vi "closeDevices.vi"(8 "Erreur d'entrée DAS":errorcluster caption="Error in", 9 "ID a l'entrée":T1, 10 "Erreur d'entrée alim":errorcluster caption="Error in", 11 "Device information in":string[](array[string])) -> (0 "Erreur de sortie":errorcluster caption="valeur sélectionnée", 1 "TCP/IP Settings:Dot-Notation Address":string)   [LabVIEW 2019]
doc: "Il ferme tous les connections avec les machines."
uses:
  <instrlib>/Sefram DAS240/Sefram DAS240.lvlib
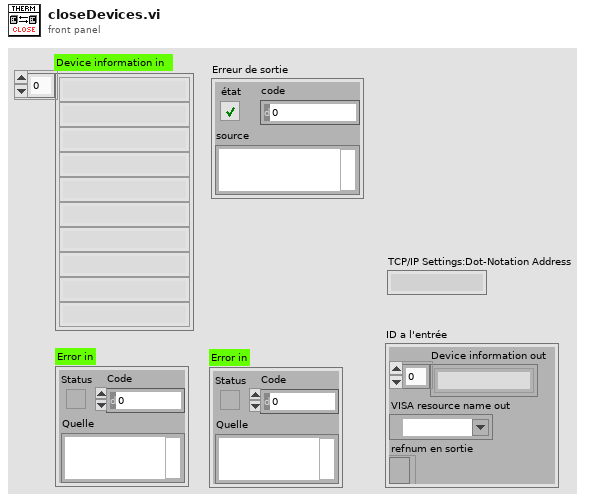
[diagram p1: front panel]
types:
  T1 = cluster{"Device information out":string[], "VISA resource name out":refnum<visa-resource-name>, "refnum en sortie":refnum<file>}
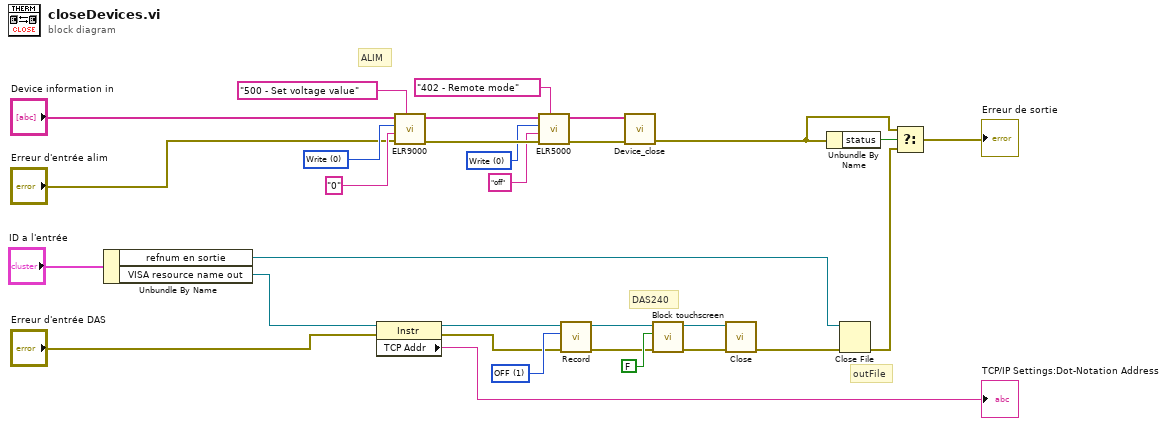
[diagram p0: block diagram]
diagram:
  w13 = u16 1 items=["ON", "OFF", "TRIG"] ("Record State")
  w21 = u8 0 items=["Write", "Read"] ("Access")
  w26 = u8 0 items=["Write", "Read"] ("Access")
  # "outFile"
  # "DAS240"
  # "ALIM"
  n1 = Unbundle By Name("ID a l'entrée") -> ("refnum en sortie"=w9:refnum<file>, "VISA resource name out"=w2:refnum<visa-resource-name>)
  n2 = property class="Instr"(reference=w2, error in="Erreur d'entrée DAS") -> (reference out=w3:refnum<visa-resource-name>, error out=w4:errorcluster, "TCP Addr"=→"TCP/IP Settings:Dot-Notation Address":string)
  n3 = call <instrlib>:"ELR9000.vi"("Command list"="500 - Set voltage value", "Error in"="Erreur d'entrée alim", "Value"="0", "Access"=w26, "Device information in"="Device information in") -> ("Error out"=w24:errorcluster, "Device information out"=w25:string[])  [unwired: 1 in, 2 out]
  n4 = call <instrlib>:"ELR5000.vi"("Command list"="402 - Remote mode", "Error in"=w24, "Value"="off", "Access"=w21, "Device information in"=w25) -> ("Error out"=w22:errorcluster, "Device information out"=w23:string[])  [unwired: 1 in, 2 out]
  n5 = call <instrlib>:"Record.vi"("error in (no error)"=w4, "Record State"=w13, "VISA resource name"=w3) -> ("error out"=w11:errorcluster, "VISA resource name out"=w12:refnum<visa-resource-name>)  [unwired: 7 in]
  n6 = call <instrlib>:"Device_close.vi"("error in (no error)"=w22, "Device information in"=w23) -> ("Fehler (Ausgang)"=w29:errorcluster)  [unwired: 3 in]
  n7 = call <instrlib>:"Block touchscreen.vi"("error in (no error)"=w11, "Block touchscreen?"=FALSE, "VISA resource name"=w12) -> ("error out"=w15:errorcluster, "VISA resource name out"=w16:refnum<visa-resource-name>)  [unwired: 7 in]
  n8 = call <instrlib>:"Close.vi"("error in (no error)"=w15, "VISA resource name"=w16) -> ("error out"=w8:errorcluster)  [unwired: 9 in]
  n9 = Unbundle By Name(w29) -> ("status"=w30:bool)
  n10 = Close File(refnum=w9, error in=w8) -> (error out=w7:errorcluster)  [unwired: 1 out]
  n11 = Select(t=w29, s=w30, f=w7) -> (s? t:f=→"Erreur de sortie":errorcluster)
